vi "Synchronized AO Generation.vi"() -> ()   [LabVIEW 2018, in "GettingStarted_5745_Host.lvlib"]
uses:
  GettingStarted_5745_Host.lvlib
  <resource>/objmgr/niflexrioapiStream.rc
  <instrlib>/FlexRIO/API/Host/v1/NI FlexRIO API v1.lvlib
  <vilib>/rvi/interface/nirviCloseFPGA/nirviCloseFPGA.xnode
  <resource>/objmgr/niflexrioapi.rc
  <instrlib>/_niInstr/Streaming/v1/Host/Public/Start Continuous Stream.vi
  <instrlib>/FlexRIO/API/Host/v1/NI FlexRIO/API/Configure Digital Edge Start Trigger.vi
  <instrlib>/FlexRIO/API/Host/v1/NI FlexRIO/API/Get Property Reference - Fpga Small.vi
  <vilib>/FPGAPlugInAG/Dynamic/niLvFpga_Close_Dynamic.vi
  <vilib>/userDefined/High Color/nirio_resource_hc.ctl
panel:
  in  "sampling info":cluster{"Fs":dbl, "#s":dbl}={"Fs"=3200000000.0, "#s"=1600.0} {"Fs" format="%#_6p"}
  in  "flexrio generators":T2(array[cluster])
  in  "amplitude":dbl=0.2 format="%0.2p"
  in  "frequency":dbl=32000000.0 format="%0.2p"
  out "generation active":bool[](array[boolean])
  in  "stop":bool
  in  "trigger source":string(combo)
  in  "trigger mode":enum16{"Immediate", "Digital"}(ring)
  out "error out":errorcluster
  out "Output Waveform":waveform(dbl)(graph)={"t0"=timestamp(0 s since 1904-01-01), "dt"=3.125e-10, "Y"=[0.0, 0.02511620781172535, 0.0501332934257217, 0.07495252583428985, 0.09947595486594193, 0.12360679774997897, 0.14724982107387122, 0.17031171662602906, 0.19270146964068613, 0.21433071799159867, 0.23511410091698928, 0.25496959589947593, 0.2738188423714755, 0.29158745096856464, 0.30820529711031575, 0.323606797749979, 0.3377311702008061, 0.3505226720175455, 0.3619308209864079, 0.3719105943553006, 0.3804226065180615, 0.3874332644514525, 0.3929149002914755, 0.3968458805257912, 0.39921069137130866, 0.4, 0.39921069137130866, 0.3968458805257912, 0.3929149002914755, 0.3874332644514525, 0.3804226065180615, 0.3719105943553006, 0.3619308209864079, 0.3505226720175455, 0.3377311702008061, 0.323606797749979, 0.3082052971103158, 0.29158745096856464, 0.2738188423714756, 0.25496959589947593, 0.23511410091698937, 0.2143307179915987, 0.1927014696406862, 0.17031171662602912, 0.14724982107387127, 0.12360679774997903, 0.09947595486594199, 0.07495252583428991, 0.05013329342572176, 0.025116207811725404, 4.85722573273506e-17, -0.0251162078117253, -0.05013329342572166, -0.0749525258342898, -0.09947595486594189, -0.12360679774997892, -0.1472498210738712, -0.170311716626029, -0.19270146964068613, -0.2143307179915986, -0.23511410091698928, -0.2549695958994759, -0.2738188423714755, -0.2915874509685646, -0.30820529711031575, -0.32360679774997897, -0.3377311702008061, -0.35052267201754544, -0.36193082098640794, -0.3719105943553006, -0.3804226065180616, -0.3874332644514525, -0.39291490029147563, -0.3968458805257912, -0.3992106913713088, -0.4, -0.3992106913713088, -0.3968458805257912, -0.3929149002914757, -0.3874332644514525, -0.38042260651806165, -0.3719105943553006, -0.36193082098640805, -0.3505226720175455, -0.3377311702008063, -0.323606797749979, -0.30820529711031597, -0.29158745096856464, -0.27381884237147575, -0.25496959589947593, -0.2351141009169895, -0.2143307179915987, -0.19270146964068635, -0.17031171662602912, -0.1472498210738714, -0.12360679774997903, -0.0994759548659421, -0.07495252583428991, -0.05013329342572185, -0.025116207811725404]}
  # "This example demonstrates how to synchronize AO streams across multiple devices.\n\nThe same waveform is downloaded to each each device, and generation will begin on AO0 and AO1 when the start trigger is received."
  # "Generation trigger configuration"
  # "Digital Trigger configuration"
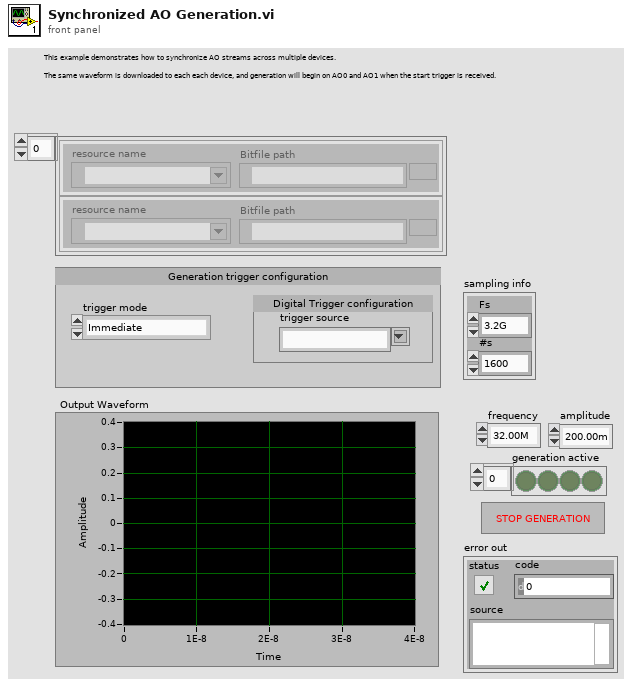
[diagram p1: front panel]
types:
  T1 = typedef "nirio_resource_hc.ctl" = tag
  T2 = cluster{"resource name":T1, "Bitfile path":path}[]
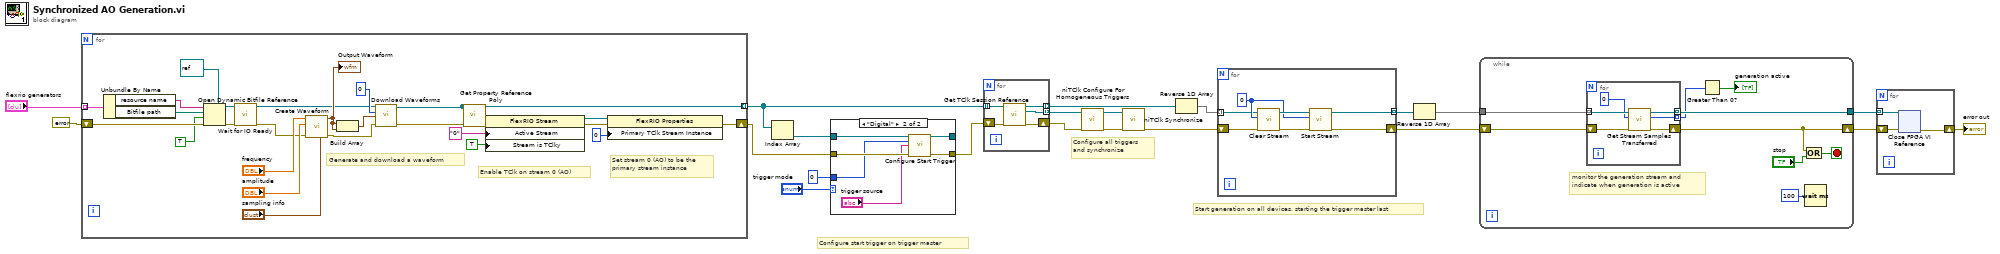
[diagram p0: block diagram]
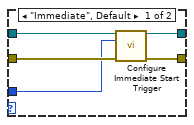
[diagram p2: hidden frame]
diagram:
  # "Configure all triggers \nand synchronize"
  # "Start generation on all devices, starting the trigger master last"
  # "Configure start trigger on trigger master"
  n1 = for {
    tunnel: "flexrio generators" -> [w28] mode=indexing
    tunnel: [w38] -> w11 mode=indexing
    shift-right: [w42] -> w13
    shift-left: errorcluster {"status"=FALSE, "code"=0, "source"=""} ("error out") -> [w39]
    # "Set stream 0 (AO) to be the\nprimary stream instance"
    # "Enable TClk on stream 0 (AO)"
    # "Generate and download a waveform"
    n2 = Unbundle By Name(w28) -> ("resource name"=w27:T1, "Bitfile path"=w26:path)
    n3 = Open Dynamic Bitfile Reference(0:w27, 1:w26, 2:TRUE ("Run When Loaded"), 3:w39, 4:refnum<k20> refnum ("FPGA VI Reference Out")) -> (5:w29:refnum<k20>, 8:w30:errorcluster)
    n4 = call <instrlib>:"Wait for IO Ready.vi"("fpga interface in"=w29, "error in"=w30) -> ("fpga interface out"=w24:refnum<k20>, "error out"=w23:errorcluster)  [unwired: 10 in, 2 out]
    n5 = call "Create Waveform.vi"("sampling info"="sampling info", "error in (no error)"=w23, "amplitude"="amplitude", "frequency"="frequency") -> ("error out"=w31:errorcluster, "Output Waveform (V)"=w35:waveform(dbl))  [unwired: 5 in, 1 out]
    "Output Waveform" <- w35
    n6 = Build Array(w35, w35) -> (w37:waveform(dbl)[])
    n7 = call "Download Waveforms.vi"("fpga interface in"=w24, "stream instance"=0, "waveforms"=w37, "error in"=w31) -> ("fpga interface out"=w38:refnum<k20>, "error out"=w33:errorcluster)  [unwired: 9 in, 1 out]
    n8 = call-poly <instrlib>:"Get Property Reference Poly.vi"("error in (no error)"=w33, "fpga interface in"=w38) -> ("error out"=w48:errorcluster, "property reference"=w47:refnum<k20>)  [unwired: 4 in, 1 out]
    n9 = property class="FlexRIO Stream"(reference=w47, error in=w48, "Active Stream"="0", "Stream is TClky"=TRUE ("Configuration:Stream is TClky")) -> (reference out=w44:refnum<k20>, error out=w43:errorcluster)
    n10 = property class="FlexRIO Properties"(reference=w44, error in=w43, "Primary TClk Stream Instance"=0 ("Device:Primary TClk Stream Instance")) -> (error out=w42:errorcluster)  [unwired: 1 out]
  }
  n11 = Index Array(array=w11) -> (element=w15:refnum<k20>)  [unwired: 1 in]
  n12 = case shown="\"Digital\"" "trigger mode" {
    tunnel: w13 -> [w53 w58]
    tunnel: w15 -> [w50 w59]
    tunnel: [w52 w57] -> w12
    tunnel: [w49 w56] -> _
    tunnel: u32 0 ("trigger instance") -> [w51 w54]
    frame "Immediate", Default {
      n13 = call <instrlib>:"Configure Immediate Start Trigger.vi"("fpga interface in"=w50, "trigger instance"=w51, "error in"=w53) -> ("fpga interface out"=w49:refnum<k20>, "error out"=w52:errorcluster)  [unwired: 10 in, 1 out]
    }
    frame "Digital" {
      n14 = call-poly <instrlib>:"Configure Start Trigger.vi"("fpga interface in"=w59, "trigger instance"=w54, "trigger source"="trigger source", "error in"=w58) -> ("fpga interface out"=w56:refnum<k20>, "error out"=w57:errorcluster)  [unwired: 9 in, 1 out]
    }
  }
  n15 = for {
    tunnel: w11 -> [w63] mode=indexing
    tunnel: [w62] -> w20 mode=indexing
    tunnel: [w61] -> w9 mode=indexing
    shift-right: [w60] -> w21
    shift-left: w12 -> [w64]
    n16 = call <instrlib>:"Get TClk Session Reference.vi"("fpga interface in"=w63, "error in"=w64) -> ("fpga interface out"=w61:refnum<k20>, "tclk session reference"=w62:refnum<k20>, "error out"=w60:errorcluster)  [unwired: 11 in]
  }
  n17 = call <instrlib>:"niTClk Configure For Homogeneous Triggers.vi"("error in (no error)"=w21, "sessions"=w20) -> ("error out"=w19:errorcluster, "sessions out"=w18:refnum<k20>[])  [unwired: 8 in]
  n18 = call <instrlib>:"niTClk Synchronize.vi"("error in (no error)"=w19, "sessions"=w18) -> ("error out"=w7:errorcluster)  [unwired: 8 in, 1 out]
  n19 = Reverse 1D Array(array=w9) -> (reversed array=w8:refnum<k20>[])
  n20 = for {
    tunnel: w8 -> [w67] mode=indexing
    shift-right: [w66] -> w6
    shift-left: w7 -> [w68]
    tunnel: [w65] -> w5 mode=indexing
    w69 = 0 ("stream index")
    n21 = call <instrlib>:"Clear Stream.vi"("error in (no error)"=w68, "stream index"=w69, "refnum in"=w67) -> ("error out"=w71:errorcluster, "refnum out"=w70:refnum<k20>)  [unwired: 7 in]
    n22 = call-poly <instrlib>:"Start Stream.vi"("error in (no error)"=w71, "stream index"=w69, "refnum in"=w70) -> ("error out"=w66:errorcluster, "refnum out"=w65:refnum<k20>)  [unwired: 7 in]
  }
  n23 = Reverse 1D Array(array=w5) -> (reversed array=w3:refnum<k20>[])
  n24 = while {
    tunnel: w3 -> [w78]
    tunnel: [w77] -> w10
    shift-right: [w72] -> w4
    shift-left: w6 -> [w73]
    stop <- w80 stop-if-true
    # "monitor the generation stream and \nindicate when generation is active"
    n25 = for {
      shift-right: [w86] -> w72
      shift-left: w73 -> [w85]
      tunnel: w78 -> [w84] mode=indexing
      tunnel: [w82] -> w77 mode=indexing
      tunnel: [w81] -> w75 mode=indexing
      n26 = call <instrlib>:"Get Stream Samples Transferred.vi"("error in (no error)"=w85, "stream index"=0, "refnum in"=w84) -> ("error out"=w86:errorcluster, "samples transferred"=w81:u64, "refnum out"=w82:refnum<k20>)  [unwired: 6 in]
    }
    n27 = Greater Than 0?(x=w75) -> (x > 0?=→"generation active":bool[])
    n28 = Or(x=w72, y="stop") -> (x .or. y?=w80:bool)
    n29 = Wait (ms)(milliseconds to wait=u32 100) -> ()  [unwired: 1 out]
  }
  n30 = for {
    tunnel: w10 -> [w88] mode=indexing
    shift-right: [w87] -> w17
    shift-left: w4 -> [w89]
    n31 = xnode "Close FPGA VI Reference"("FPGA VI Reference In"=w88, "error in"=w89) -> ("error out"=w87:errorcluster)
  }
  "error out" <- w17
